vi "Logger DSC Sandbox.vi"() -> ()   [LabVIEW 2019]
uses:
  <resource>/objmgr/ni.var.rc
  <vilib>/JKI/JKI SMO/URI Parsing/URI.lvlib
  <vilib>/lvdsc/NI_DSC.lvlib
panel:
  out "error out 3":errorcluster
  out "error out 2":errorcluster
  out "URI":string
  out "error out":errorcluster
  out "Writable":bool
  out "URL":string
  out "Readable":bool
  out "Parent":refnum<k21>
  out "Name":string
  out "Engine":refnum<k21>
  out "Class Identifier":string
  in  "variable name":string
  in  "process name":string="JLevy"
  # "SR7270_09337296"
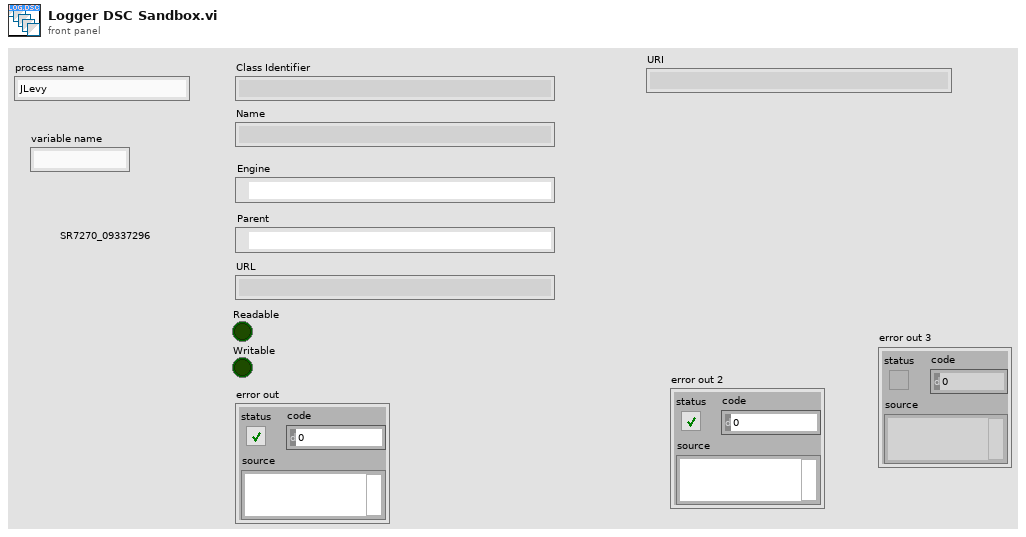
[diagram p1: front panel]
types:
  T1 = enum32{"u32BitField", "bool", "double", "string", "int8", "uint8", "int16", "uint16", "int32", "uint32", "int64", "uint64", "single", "double waveform", "int16 waveform", "array of boolean", "array of int8", "array of uint8", "array of int16", "array of uint16", "array of int32", "array of uint32", "array of int64", "array of uint64", "array of single", "array of double", "array of double waveform", "array of int16 waveform", "array of string", "variant", "timestamp", "fixed point", "custom"}
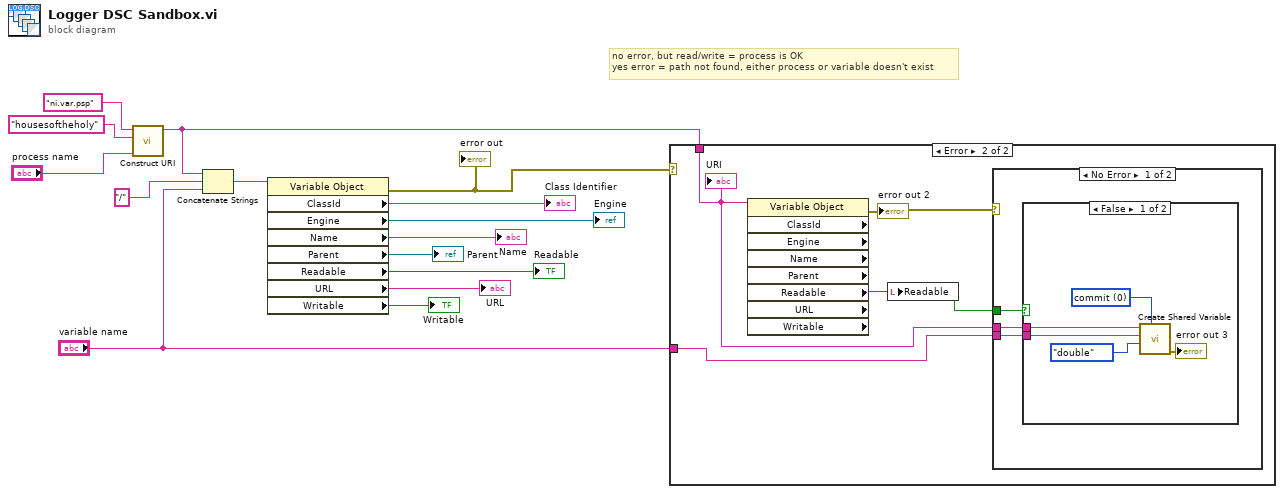
[diagram p0: block diagram]
diagram:
  # "no error, but read/write = process is OK\nyes error = path not found, either process or variable doesn't exist"
  n1 = call <vilib>:"Construct URI.vi"("path"="process name", "address"="housesoftheholy", "protocol"="ni.var.psp") -> ("URI"=w1:string)  [unwired: 8 in]
  n2 = Concatenate Strings(w1, "/" ("string"), "variable name") -> (w3:string)
  n3 = property class="Variable Object"(reference=w3) -> (error out=w5:errorcluster, "ClassId"=→"Class Identifier":string, "Engine"=→"Engine":refnum<k21>, "Name"=→"Name":string, "Parent"=→"Parent":refnum<k21>, "Readable"=→"Readable":bool, "URL"=→"URL":string, "Writable"=→"Writable":bool)  [unwired: 1 in, 1 out]
  "error out" <- w5
  n4 = case shown="Error" w5 {
    tunnel: "variable name" -> [_ w16]
    tunnel: w1 -> [_ w17]
    frame No Error {
    }
    frame Error {
      n5 = property class="Variable Object" props=["ClassId", "Engine", "Name", "Parent", "Readable", "URL", "Writable"](reference=w17) -> (error out=w19:errorcluster, "Readable"=w18:bool)  [unwired: 1 in, 7 out]
      "error out 2" <- w19
      n6 = local write "Readable"(w18) -> ()
      n7 = case shown="No Error" w19 {
        tunnel: w18 -> [w22 _]
        tunnel: w17 -> [w21 _]
        tunnel: w16 -> [w20 _]
        frame No Error {
          n8 = case shown="False" w22 {
            tunnel: w21 -> [w27 _]
            tunnel: w20 -> [w25 _]
            frame False {
              w26 = u16 0 items=["commit", "buffer"] ("set mode")
              n9 = call <vilib>:"Create Shared Variable.vi"("set mode"=w26, "data type"=T1."double", "shared variable name"=w25, "process name"=w27) -> ("error out"=→"error out 3":errorcluster)  [unwired: 5 in, 2 out]
            }
            frame True {
            }
          }
        }
        frame Error {
        }
      }
      "URI" <- w17
    }
  }
